vi "SVL Initialize Waterfall Display.vi"(0 "window title":string="Waterfall", 5 "display bounds":T2={"left"=20, "top"=20, "width"=600, "height"=400} {"height" min=300; "width" min=400}, 7 "number of plots":i32, 11 "error in (no error)":errorcluster, 12 "colors":T1={"frame"=16763904, "plot"=52224, "background"=0}) -> (4 "waterfall ref":refnum<vi>, 15 "error out":errorcluster)   [LabVIEW 2017]
doc: "Initializes the waterfall display and generates the waterfall reference used to send data to the display or to close the display."
uses:
  <vilib>/addons/Sound and Vibration/compatibility/Waterfall/subVIs/svl_Waterfall Global.vi
panel:
  in  "invalid waterfall ref":refnum<vi>
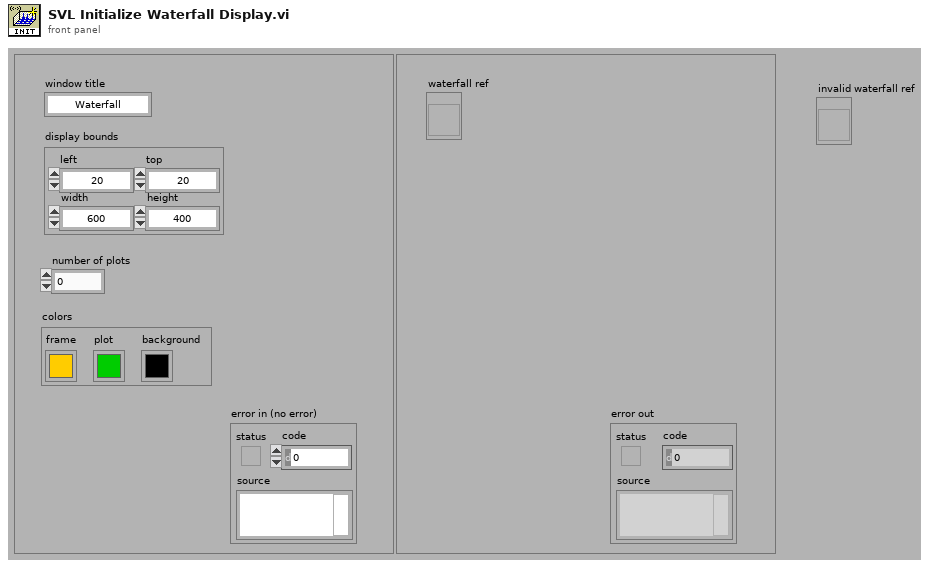
[diagram p1: front panel]
types:
  T1 = cluster{"frame":u32, "plot":u32, "background":u32}
  T2 = cluster{"left":i16, "top":i16, "width":i16, "height":i16}
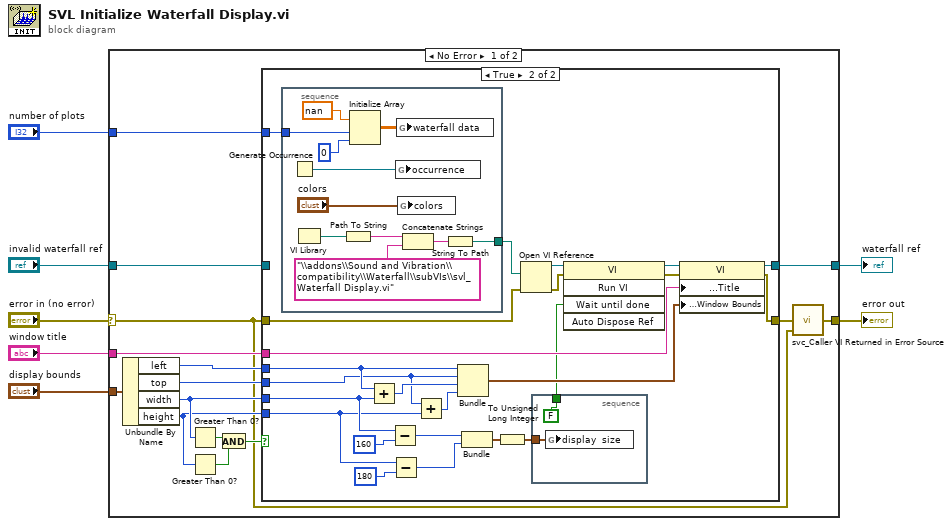
[diagram p0: block diagram]
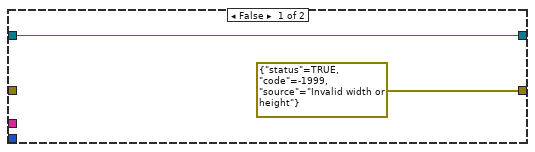
[diagram p2: hidden frame]
diagram:
  n1 = case shown="No Error" "error in (no error)" {
    selector: "error in (no error)" -> [w8 w63]
    tunnel: [w19 w63] -> w7
    tunnel: [w12 w62] -> w6
    tunnel: "window title" -> [w18 _]
    tunnel: "display bounds" -> [w17 _]
    tunnel: "invalid waterfall ref" -> [w10 w62]
    tunnel: "number of plots" -> [w9 _]
    frame No Error {
      n2 = Unbundle By Name(w17) -> ("left"=w21:i16, "top"=w20:i16, "width"=w16:i16, "height"=w15:i16)
      n3 = Greater Than 0?(x=w16) -> (x > 0?=w14:bool)
      n4 = Greater Than 0?(x=w15) -> (x > 0?=w13:bool)
      n5 = And(x=w14, y=w13) -> (x .and. y?=w11:bool)
      n6 = case shown="True" w11 {
        tunnel: [errorcluster {"status"=TRUE, "code"=-1999, "source"="Invalid width or height"} ("Error IO") w48] -> w22
        tunnel: w21 -> [_ w46]
        tunnel: w20 -> [_ w44]
        tunnel: [w23 w36] -> w12
        tunnel: w8 -> [_ w26]
        tunnel: w18 -> [_ w30]
        tunnel: w16 -> [_ w29]
        tunnel: w15 -> [_ w28]
        tunnel: w10 -> [w23 _]
        tunnel: w9 -> [_ w25]
        frame False {
        }
        frame True {
          n7 = stacked-sequence {
            tunnel: [w54] -> w31
            tunnel: w25 -> [w49]
            frame #0 {
              n8 = Generate Occurrence() -> (w58:refnum<k4>)
              n9 = VI Library() -> (path=w57:path)
              n10 = Path To String(path=w57) -> (string=w55:string)
              n11 = Initialize Array(nan ("element"), w49, 0 ("dimension size")) -> (w50:dbl[][])
              n12 = global write "svl_Waterfall Global.vi" "occurrence"(w58) -> ()
              n13 = global write "svl_Waterfall Global.vi" "waterfall data"(w50) -> ()
              n14 = global write "svl_Waterfall Global.vi" "colors"("colors") -> ()
              n15 = Concatenate Strings(w55, "\\addons\\Sound and Vibration\\compatibility\\Waterfall\\subVIs\\svl_Waterfall Display.vi" ("Substring")) -> (w56:string)
              n16 = String To Path(string=w56) -> (path=w54:path)
            }
          }
          n17 = Add(x=w46, y=w29) -> (x+y=w45:i16)
          n18 = Subtract(x=w29, y=i16 160) -> (x-y=w39:i16)
          n19 = Subtract(x=w28, y=i16 180) -> (x-y=w37:i16)
          n20 = Add(x=w44, y=w28) -> (x+y=w43:i16)
          n21 = Bundle("left"=w46, "top"=w44, w45, w43) -> (w47:cluster{"left":i16, "top":i16, i16, i16})  [unwired: 1 in]
          n22 = Bundle(w39, w37) -> (w42:cluster{i16, i16})  [unwired: 1 in]
          n23 = To Unsigned Long Integer(number=w42) -> (unsigned 32bit integer=w41:cluster{u32, u32})
          n24 = Open VI Reference(vi path=w31, error in (no error)=w26) -> (vi reference=w32:refnum<vi>, error out=w33:errorcluster)  [unwired: 4 in]
          n25 = stacked-sequence {
            tunnel: w41 -> [w61]
            tunnel: [FALSE ("Wait until done")] -> w27
            frame #0 {
              n26 = global write "svl_Waterfall Global.vi" "display  size"(w61) -> ()
            }
          }
          n27 = invoke class="VI" method="Run VI"(reference=w32, error in=w33, "Wait until done"=w27) -> (reference out=w34:refnum<vi>, error out=w35:errorcluster)  [unwired: 2 in, 3 out]
          n28 = property class="VI"(reference=w34, error in=w35, "Front Panel Window:Title"=w30, "Front Panel Window:Window Bounds"=w47) -> (reference out=w36:refnum<vi>, error out=w48:errorcluster)
        }
      }
      n29 = call <vilib>:"svc_Caller VI Returned in Error Source.vi"("warning input to caller"=w8, "error in (no error)"=w22) -> ("error out"=w19:errorcluster)  [unwired: 3 in]
    }
    frame Error {
    }
  }
  "error out" <- w7
  "waterfall ref" <- w6
